vi "GoToBallSkillVSS.vi"(7 "First call?":bool=TRUE, 8 "error in (no error)":errorcluster, 9 "Game":refnum<class "Game.lvclass">, 10 "Robot in":refnum<class "Robot.lvclass">, 11 "GoToBallSkillVSS in":refnum<class "GoToBallSkillVSS.lvclass">) -> (0 "error out":errorcluster, 1 "Robot out":refnum<class "Robot.lvclass">, 3 "GoToBallSkillVSS out":refnum<class "GoToBallSkillVSS.lvclass">)   [LabVIEW 2020, in "GoToBallSkillVSS.lvclass"]
uses:
  GoToBallSkillVSS.lvclass
  Robot_class/Robot.lvclass
  C:/Users/lucio/Desktop/Horie/ROBOIME/VSS_AI/Object_class/Object.lvclass
  Game_class/Game.lvclass
  Object_class/Object.lvclass/Object.ctl
  Robot_class/Robot.lvclass/Robot.ctl
  Game_class/Game.lvclass/Game.ctl
  Robot_class/stateGotoballskill.ctl
  Game_class/Read FieldRef.vi
  Game_class/Read BallRef.vi
  Object_class/Read x.vi
  Object_class/Read y.vi
  Robot_class/Read orientation.vi
  Robot_class/Write dest_orientation.vi
  Robot_class/Write dest_x.vi
  Robot_class/Write dest_y.vi
  Ball_class/Ball.lvclass
  Field_class/Field.lvclass
panel:
  in  "SideballY 2":dbl=-120.0
  in  "SideballX":dbl=50.0
  in  "SideballY":dbl=-120.0
  in  "Behindball":dbl=50.0
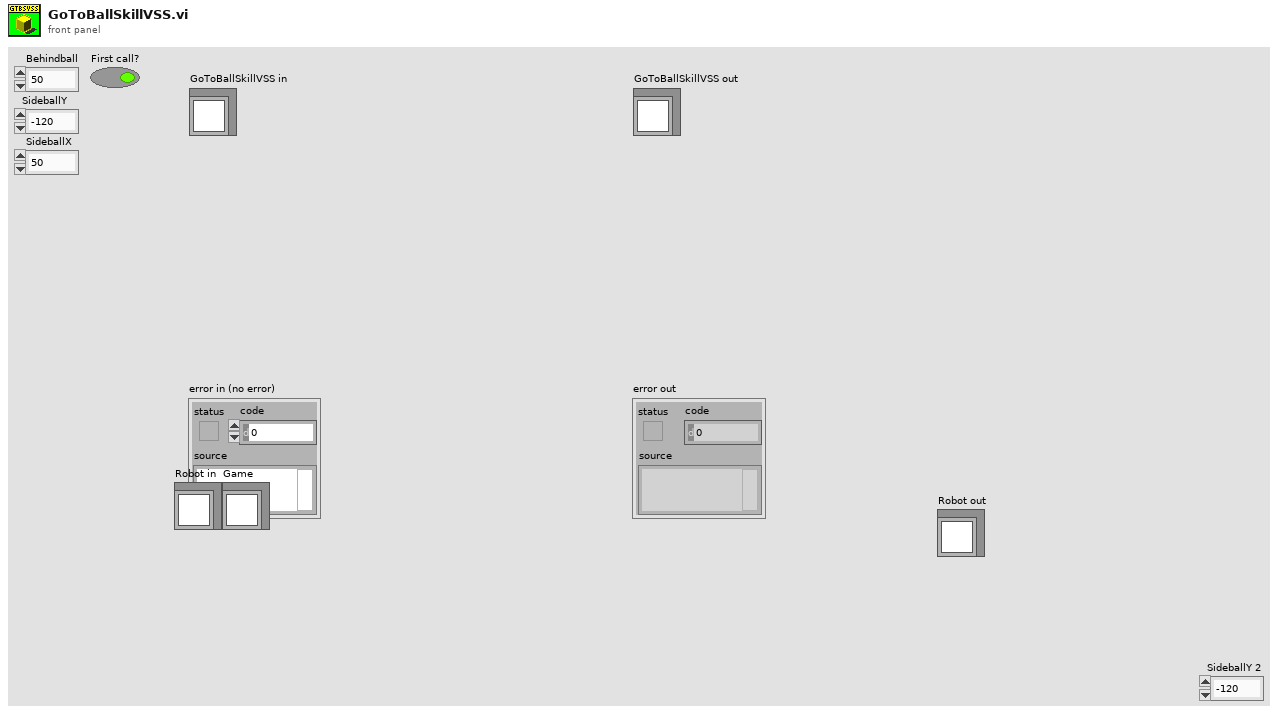
[diagram p1: front panel]
types:
  T1 = typedef "stateGotoballskill.ctl" = enum16{"Indobola", "Indoatras", "Indolateral"}
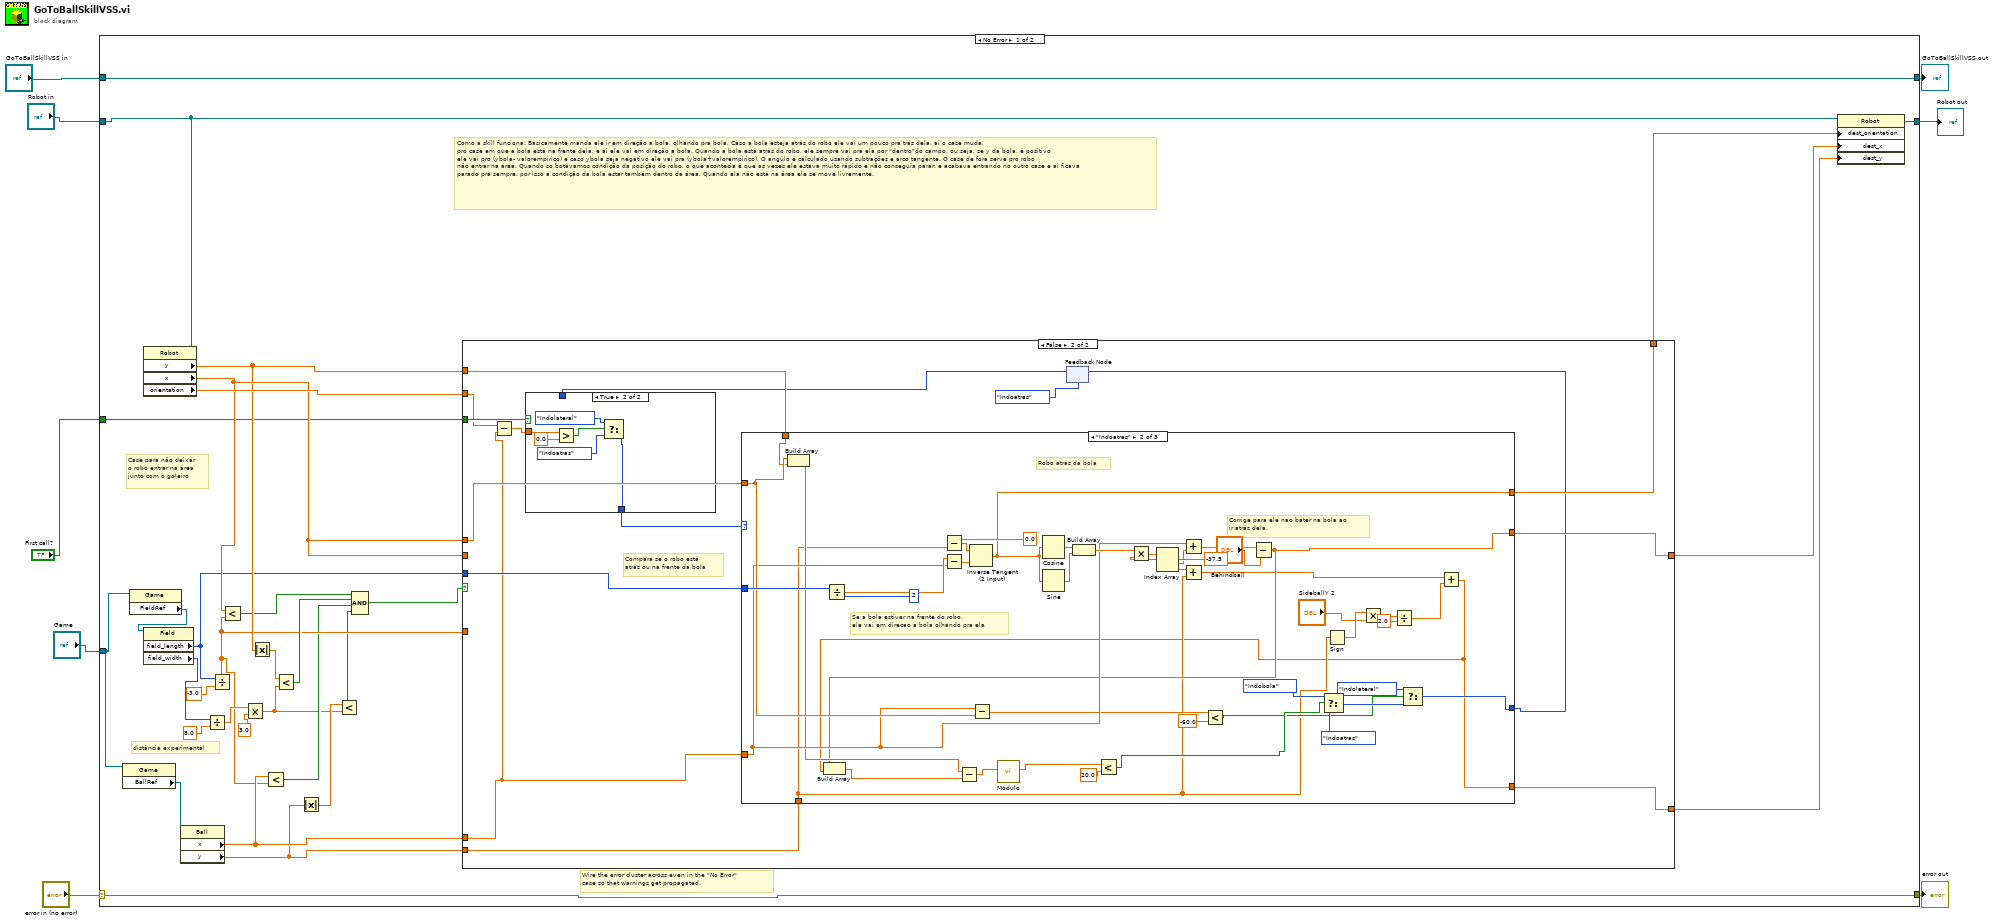
[diagram p0: block diagram]
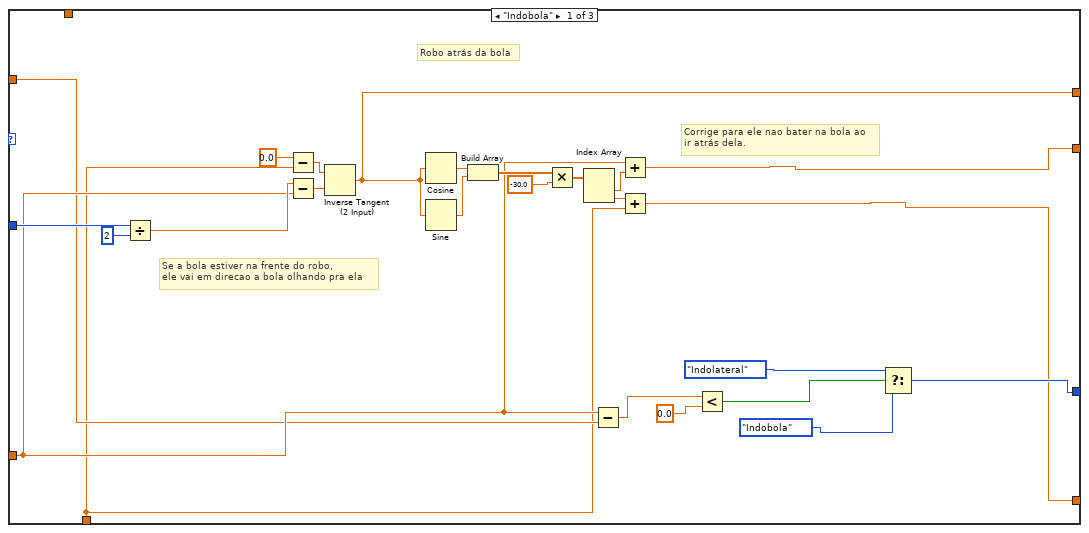
[diagram p4: hidden frame]
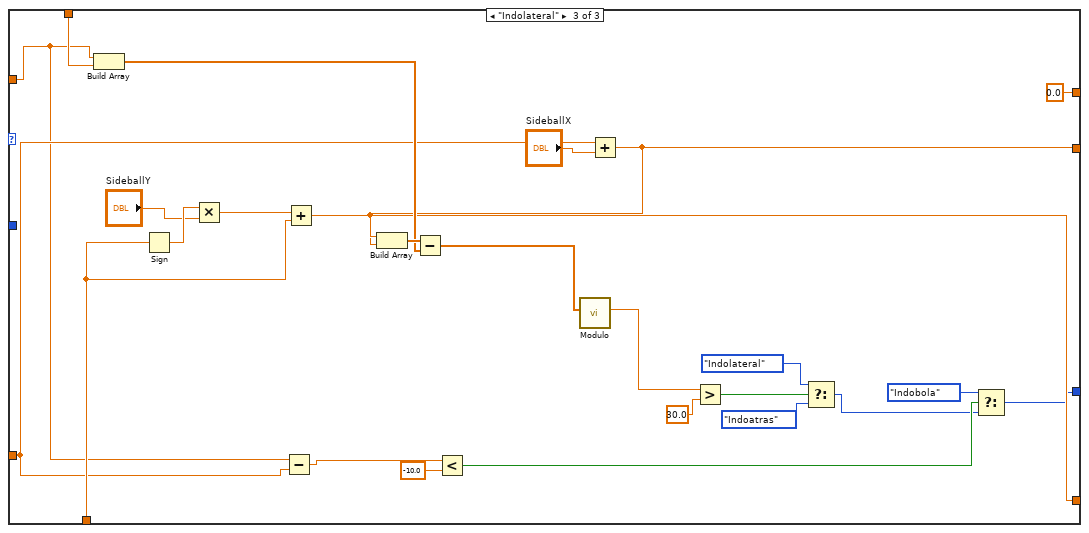
[diagram p5: hidden frame]
diagram:
  n1 = case shown="No Error" "error in (no error)" {
    selector: "error in (no error)" -> [w38 w159]
    tunnel: [w38 w159] -> w7
    tunnel: [w39 w158] -> w5
    tunnel: "GoToBallSkillVSS in" -> [w39 w158]
    tunnel: [w35 w157] -> w3
    tunnel: "Robot in" -> [w34 w157]
    tunnel: "Game" -> [w31 _]
    tunnel: "First call?" -> [w9 _]
    frame No Error {
      # "Como a skill funciona: Basicamente manda ele ir em direção a bola, olhando pra bola. Caso a bola esteja atrás do robo ele vai um pouco pra trás dela, ai o case muda,\npro case em que a bola está na frente dela, e ai ele vai em direção a bola. Quando a bola está atrás do robo, ele sempre vai pra ela por \"dentro\"do campo, ou seja, se y da bola, é positivo\nele vai pro (ybola- valorempirico) e caso ybola seja negativo ele vai pra (ybola+valorempirico). O angulo é calculado usando subtrações e arco tangente. O case de fora serve pro robo\nnão entrar na área. Quando so botávamos condição da posição do robo, o que acontecia é que as vezes ele estava muito rápido e não conseguia parar, e acabava entrando no outro case e ai ficava parado pra sempre, por isso a condição da bola estar também dentro da área. Quando ela não está na área ele se move livremente."
      # "distância experimental"
      # "Case para não deixar\no robo entrar na área\njunto com o goleiro"
      # "Wire the error cluster across even in the \"No Error\"\ncase so that warnings get propagated."
      n2 = property class="Game"(reference=w31) -> ("BallRef"=w33:refnum<class "Ball.lvclass">)  [unwired: 1 in, 2 out]
      n3 = property class="Game"(reference=w31) -> ("FieldRef"=w30:refnum<class "Field.lvclass">)  [unwired: 1 in, 2 out]
      n4 = property class="Robot"(reference=w34) -> ("y"=w25:dbl, "x"=w28:dbl, "orientation"=w29:dbl)  [unwired: 1 in, 2 out]
      n5 = property class="Field"(reference=w30) -> ("field_length"=w10:i32, "field_width"=w26:i32)  [unwired: 1 in, 2 out]
      n6 = property class="Ball"(reference=w33) -> ("x"=w18:dbl, "y"=w14:dbl)  [unwired: 1 in, 2 out]
      n7 = Divide(x=w26, y=8.0) -> (x/y=w22:dbl)
      n8 = Divide(x=w10, y=-3.0) -> (x/y=w17:dbl)
      n9 = Less?(x=w28, y=w17) -> (x < y?=w20:bool)
      n10 = Multiply(x=w22, y=3.0) -> (x*y=w13:dbl)
      n11 = Absolute Value(x=w25) -> (abs(x)=w24:dbl)
      n12 = Less?(x=w18, y=w17) -> (x < y?=w16:bool)
      n13 = Less?(x=w24, y=w13) -> (x < y?=w19:bool)
      n14 = Absolute Value(x=w14) -> (abs(x)=w15:dbl)
      n15 = Less?(x=w15, y=w13) -> (x < y?=w12:bool)
      n16 = Compound Arithmetic op=AND(w20, w19, w16, w12) -> (w11:bool)
      n17 = case shown="False" w11 {
        tunnel: w25 -> [w42 w57]
        tunnel: w28 -> [_ w52]
        tunnel: [w41 w56] -> w37
        tunnel: [w42 w55] -> w36
        tunnel: w18 -> [_ w43]
        tunnel: w14 -> [_ w54]
        tunnel: [w40 w53] -> w32
        tunnel: w28 -> [w40 _]
        tunnel: w29 -> [w41 w44]
        tunnel: w17 -> [_ _]
        tunnel: w10 -> [_ w51]
        tunnel: w9 -> [_ w48]
        frame True {
          # "Xrobot < -FL/3\ne\n|Yrobot| <3*(FW/8)\ne\n\nXball < FL/-3\ne\n|Yball|< 3*FW/8"
          # "Se ele estiver perto da area ele fica parado"
        }
        frame False {
          # "Compara se o robo está\natrás ou na frente da bola"
          n18 = Subtract(x=w44, y=w43) -> (x-y=w45:dbl)
          n19 = feedback #1(stateGotoballskill."Indoatras" ("State")) -> (w47:T1)
          n20 = case shown="True" w48 {
            tunnel: w47 -> [w58 _]
            tunnel: [w58 w61] -> w46
            tunnel: w45 -> [_ w64]
            frame False {
            }
            frame True {
              n21 = Greater?(x=w64, y=0.0) -> (0:w62:bool)
              n22 = Select(t=stateGotoballskill."Indolateral" ("State"), s=w62, f=stateGotoballskill."Indoatras" ("State")) -> (s? t:f=w61:T1)
            }
          }
          n23 = case shown="\"Indoatras\"" w46 {
            tunnel: [w76 w118 0.0] -> w56
            tunnel: w57 -> [_ w113 w153]
            tunnel: w54 -> [w66 w91 w152]
            tunnel: w43 -> [w69 w112 w139]
            tunnel: w52 -> [w67 w114 w138]
            tunnel: [w65 w90 w140] -> w55
            tunnel: [w75 w98 w141] -> w53
            tunnel: w51 -> [w80 w122 _]
            tunnel: [w71 w102 w132] -> w49
            frame "Indobola" {
              # "Corrige para ele nao bater na bola ao\nir atrás dela."
              # "Robo atrás da bola"
              # "Se a bola estiver na frente do robo, \nele vai em direcao a bola olhando pra ela"
              n24 = Divide(x=w80, y=2) -> (x/y=w78:dbl)
              n25 = Subtract(x=0.0, y=w66) -> (x-y=w88:dbl)
              n26 = Subtract(x=w78, y=w69) -> (x-y=w89:dbl)
              n27 = Inverse Tangent (2 Input)(1:w89, 2:w88) -> (0:w76:dbl)
              n28 = Cosine(x=w76) -> (cos(x)=w87:dbl)
              n29 = Sine(x=w76) -> (sin(x)=w86:dbl)
              n30 = Build Array(w87, w86) -> (w85:dbl[])
              n31 = Multiply(x=w85, y=-30.0) -> (x*y=w84:dbl[])
              n32 = Index Array(array=w84) -> (element #1=w82:dbl, element #2=w81:dbl)  [unwired: 2 in]
              n33 = Subtract(x=w69, y=w67) -> (x-y=w74:dbl)
              n34 = Add(x=w69, y=w82) -> (x+y=w75:dbl)
              n35 = Add(x=w81, y=w66) -> (x+y=w65:dbl)
              n36 = Less?(x=w74, y=0.0) -> (x < y?=w72:bool)
              n37 = Select(t=stateGotoballskill."Indolateral" ("State"), s=w72, f=stateGotoballskill."Indobola" ("State")) -> (s? t:f=w71:T1)
            }
            frame "Indoatras" {
              # "Corrige para ele nao bater na bola ao\nir atrás dela."
              # "Robo atrás da bola"
              # "Se a bola estiver na frente do robo, \nele vai em direcao a bola olhando pra ela"
              n38 = Build Array(w114, w113) -> (w110:dbl[])
              n39 = Divide(x=w122, y=2) -> (x/y=w120:dbl)
              n40 = Subtract(x=0.0, y=w91) -> (x-y=w130:dbl)
              n41 = Subtract(x=w120, y=w112) -> (x-y=w131:dbl)
              n42 = Inverse Tangent (2 Input)(1:w131, 2:w130) -> (0:w118:dbl)
              n43 = Subtract(x=w112, y=w114) -> (x-y=w101:dbl)
              n44 = Cosine(x=w118) -> (cos(x)=w129:dbl)
              n45 = Sine(x=w118) -> (sin(x)=w128:dbl)
              n46 = Build Array(w129, w128) -> (w127:dbl[])
              n47 = Multiply(x=w127, y=-37.5) -> (x*y=w126:dbl[])
              n48 = Index Array(array=w126) -> (element #1=w124:dbl, element #2=w123:dbl)  [unwired: 2 in]
              n49 = Add(x=w112, y=w124) -> (x+y=w115:dbl)
              n50 = Add(x=w123, y=w91) -> (x+y=w92:dbl)
              n51 = Less?(x=w101, y=-60.0) -> (x < y?=w99:bool)
              n52 = Subtract(x=w115, y="Behindball") -> (x-y=w98:dbl)
              n53 = Sign(1:w91) -> (0:w97:dbl)
              n54 = Multiply(x=w97, y="SideballY 2") -> (x*y=w95:dbl)
              n55 = Divide(x=w95, y=2.0) -> (x/y=w93:dbl)
              n56 = Add(x=w92, y=w93) -> (x+y=w90:dbl)
              n57 = Build Array(w98, w90) -> (w111:dbl[])
              n58 = Subtract(x=w110, y=w111) -> (x-y=w109:dbl[])
              n59 = call "Modulo.vi"("2D vector"=w109) -> ("Modulo"=w108:dbl)  [unwired: 10 in]
              n60 = Less?(x=w108, y=20.0) -> (x < y?=w105:bool)
              n61 = Select(t=stateGotoballskill."Indobola" ("State"), s=w105, f=stateGotoballskill."Indoatras" ("State")) -> (s? t:f=w104:T1)
              n62 = Select(t=stateGotoballskill."Indolateral", s=w99, f=w104) -> (s? t:f=w102:T1)
            }
            frame "Indolateral" {
              n63 = Build Array(w138, w153) -> (w145:dbl[])
              n64 = Sign(1:w152) -> (0:w156:dbl)
              n65 = Multiply(x=w156, y="SideballY") -> (x*y=w155:dbl)
              n66 = Subtract(x=w138, y=w139) -> (x-y=w137:dbl)
              n67 = Add(x=w155, y=w152) -> (x+y=w140:dbl)
              n68 = Less?(x=w137, y=-10.0) -> (x < y?=w135:bool)
              n69 = Add(x=w139, y="SideballX") -> (x+y=w141:dbl)
              n70 = Build Array(w141, w140) -> (w146:dbl[])
              n71 = Subtract(x=w146, y=w145) -> (x-y=w142:dbl[])
              n72 = call "Modulo.vi"("2D vector"=w142) -> ("Modulo"=w144:dbl)  [unwired: 10 in]
              n73 = Greater?(x=w144, y=30.0) -> (0:w151:bool)
              n74 = Select(t=stateGotoballskill."Indolateral" ("State"), s=w151, f=stateGotoballskill."Indoatras" ("State")) -> (s? t:f=w134:T1)
              n75 = Select(t=stateGotoballskill."Indobola", s=w135, f=w134) -> (s? t:f=w132:T1)
            }
          }
          n76 = feedback-in #1(w49) -> ()
        }
      }
      n77 = property class="Robot"(reference=w34, "dest_orientation"=w37, "dest_x"=w32, "dest_y"=w36) -> (reference out=w35:refnum<class "Robot.lvclass">)  [unwired: 1 in, 1 out]
    }
    frame Error {
    }
  }
  "error out" <- w7
  "GoToBallSkillVSS out" <- w5
  "Robot out" <- w3
